vi "Navigation_Main_r1.1(new math for dist calc).vi"() -> ()   [LabVIEW 2015]
uses:
  <vilib>/myRIO/Common/Instrument Driver Framework/Utilities/typedefs/Generic FPGA Reference.ctl
  <vilib>/myRIO/Common/Instrument Driver Framework/Utilities/typedefs/myRIO v1.0 Reference.ctl
  <vilib>/myRIO/Common/Instrument Driver Framework/Utilities/typedefs/Hardware Version Enum.ctl
  <vilib>/myRIO/Common/Instrument Driver Framework/Utilities/typedefs/myRIO Generic Hardware Reference.ctl
  <vilib>/userdefined/High Color/nirio_resource_hc.ctl
  <vilib>/myRIO/Instrument Drivers/Onboard IO/PWM/typedefs/PWM Configuration.ctl
  <vilib>/myRIO/Instrument Drivers/Onboard IO/PWM/PWM.lvlib
  <vilib>/myRIO/Common/Instrument Driver Framework/myRIO v1.0/PWM/typedefs/PWM Channels Enum.ctl
  <vilib>/myRIO/Instrument Drivers/Onboard IO/PWM/typedefs/PWM Reference.ctl
  <vilib>/myRIO/Instrument Drivers/Onboard IO/PWM/vis/myRIO PWM Open.xnode
  <vilib>/myRIO/Common/Instrument Driver Framework/myRIO v1.0/PWM/vis/myRIO v1.1 Open PWM.vi
  <vilib>/rvi/interface/nirviOpenFPGA/nirviOpenFPGA.xnode
  <vilib>/myRIO/Instrument Drivers/Utilities/Utilities.lvlib
  <vilib>/rvi/interface/nirviReadWriteControl/nirviReadWriteControl.xnode
  NiFpgaLv.dll
  <vilib>/Utility/error.llb/Error Cluster From Error Code.vi
  <vilib>/rvi/interface/Simulation/niFpgaSimulationCallBeginRW.vi
  <vilib>/rvi/errors/niLvFpgaAdjustHostInterfaceError.vi
  Navi/E/FPGA Bitfiles/NavigationProjec_FPGATarget2_FPGAMainNavigati_PWPHW8gwDxI.lvbitx
  <vilib>/FPGAPlugInAG/myRIO-1900/niLvFpga_Open_myRIO-1900.vi
  <vilib>/rvi/interface/common/dynamic/niFpgaDynamicAddResources.vi
panel:
  out "x traveled":dbl
  out "x position camera":dbl
  out "x delta":dbl
  out "total":dbl
  out "step":dbl
  out "loc_flag":bool
  out "loc_x":dbl
  out "max v":dbl
  out "v left wheel":dbl
  out "v right wheel":dbl
  out "Phi desired":dbl
  out "Omega":dbl format="%.2f"
  in  "Goal Position Y":dbl=5.0
  out "x traveled":dbl
  out "y position":dbl
  out "Scale":dbl=1.0
  out "Reset X Y":dbl
  out "Desired Velocity":dbl
  out "track width(ft)":dbl=4.0
  out "phi current":dbl
  out "robot desired velocity x component\n u1 (ft/s)":dbl
  out "robot desired velocity y component\n u2 (ft/s)":dbl
  out "RM Distance (ft)":dbl
  out "RR Distance (ft)":dbl
  out "LF Distance (ft)":dbl
  out "LM Distance (ft)":dbl
  out "RF Distance (ft)":dbl
  out "LR Distance (ft)":dbl
  out "Tick Count(mSec) 2":u32 caption="Tick Count(mSec)"
  out "Right Setpoint":dbl
  out "Left Setpoint":dbl
  in  "Start Position Y":dbl=5.0
  in  "Goal Position X":dbl=5.0
  in  "Start Position X":dbl=1.0
  in  "All Stop":bool
  in  "Left Side PID Gains":T1={"proportional gain (Kc)"=0.002, "integral time (Ti, min)"=7e-07, "derivative time (Td, min)"=0.0} {"derivative time (Td, min)" format="%.8f"; "integral time (Ti, min)" format="%.8f"; "proportional gain (Kc)" format="%.8f"}
  in  "Left Side Output Range":cluster{"output high":dbl, "output low":dbl}={"output high"=0.13333, "output low"=-0.13333} {"output low" format="%.5f"; "output high" format="%.5f"}
  in  "Right Side PID Gains":T1={"proportional gain (Kc)"=0.002, "integral time (Ti, min)"=7e-07, "derivative time (Td, min)"=0.0} {"derivative time (Td, min)" format="%.8f"; "integral time (Ti, min)" format="%.8f"; "proportional gain (Kc)" format="%.8f"}
  in  "Right Side Output Range":cluster{"output high":dbl, "output low":dbl}={"output high"=0.13333, "output low"=-0.13333} {"output low" format="%.5f"; "output high" format="%.5f"}
  out "Left PWM":dbl
  out "Right PWM":dbl
  out "LF Rot Velocity (rot/s)":dbl
  out "LM Rot Velocity (rot/s)":dbl
  out "LR Rot Velocity (rot/s)":dbl
  out "RR Rot Velocity (rot/s)":dbl
  out "RM Linear Velocity (rot/s)":dbl
  out "RF Linear Velocity (rot/s)":dbl
  in  "Encoder Reset":bool
  out "SYS.SELECTA":u8 format="%08b"
  out "ENC.B_c.CNTR":i32
  out "ENC.B_b.CNTR":i32
  out "ENC.B_a.CNTR":i32
  out "ENC.A_c.CNTR":i32
  out "ENC.A_b.CNTR":i32
  out "ENC.A_a.CNTR":i32
  out "Current Rot Velocity (rot/s)":T2(graph)
  # "Motor Control Parameters"
  # "Press Go when Start and Goal Are Set"
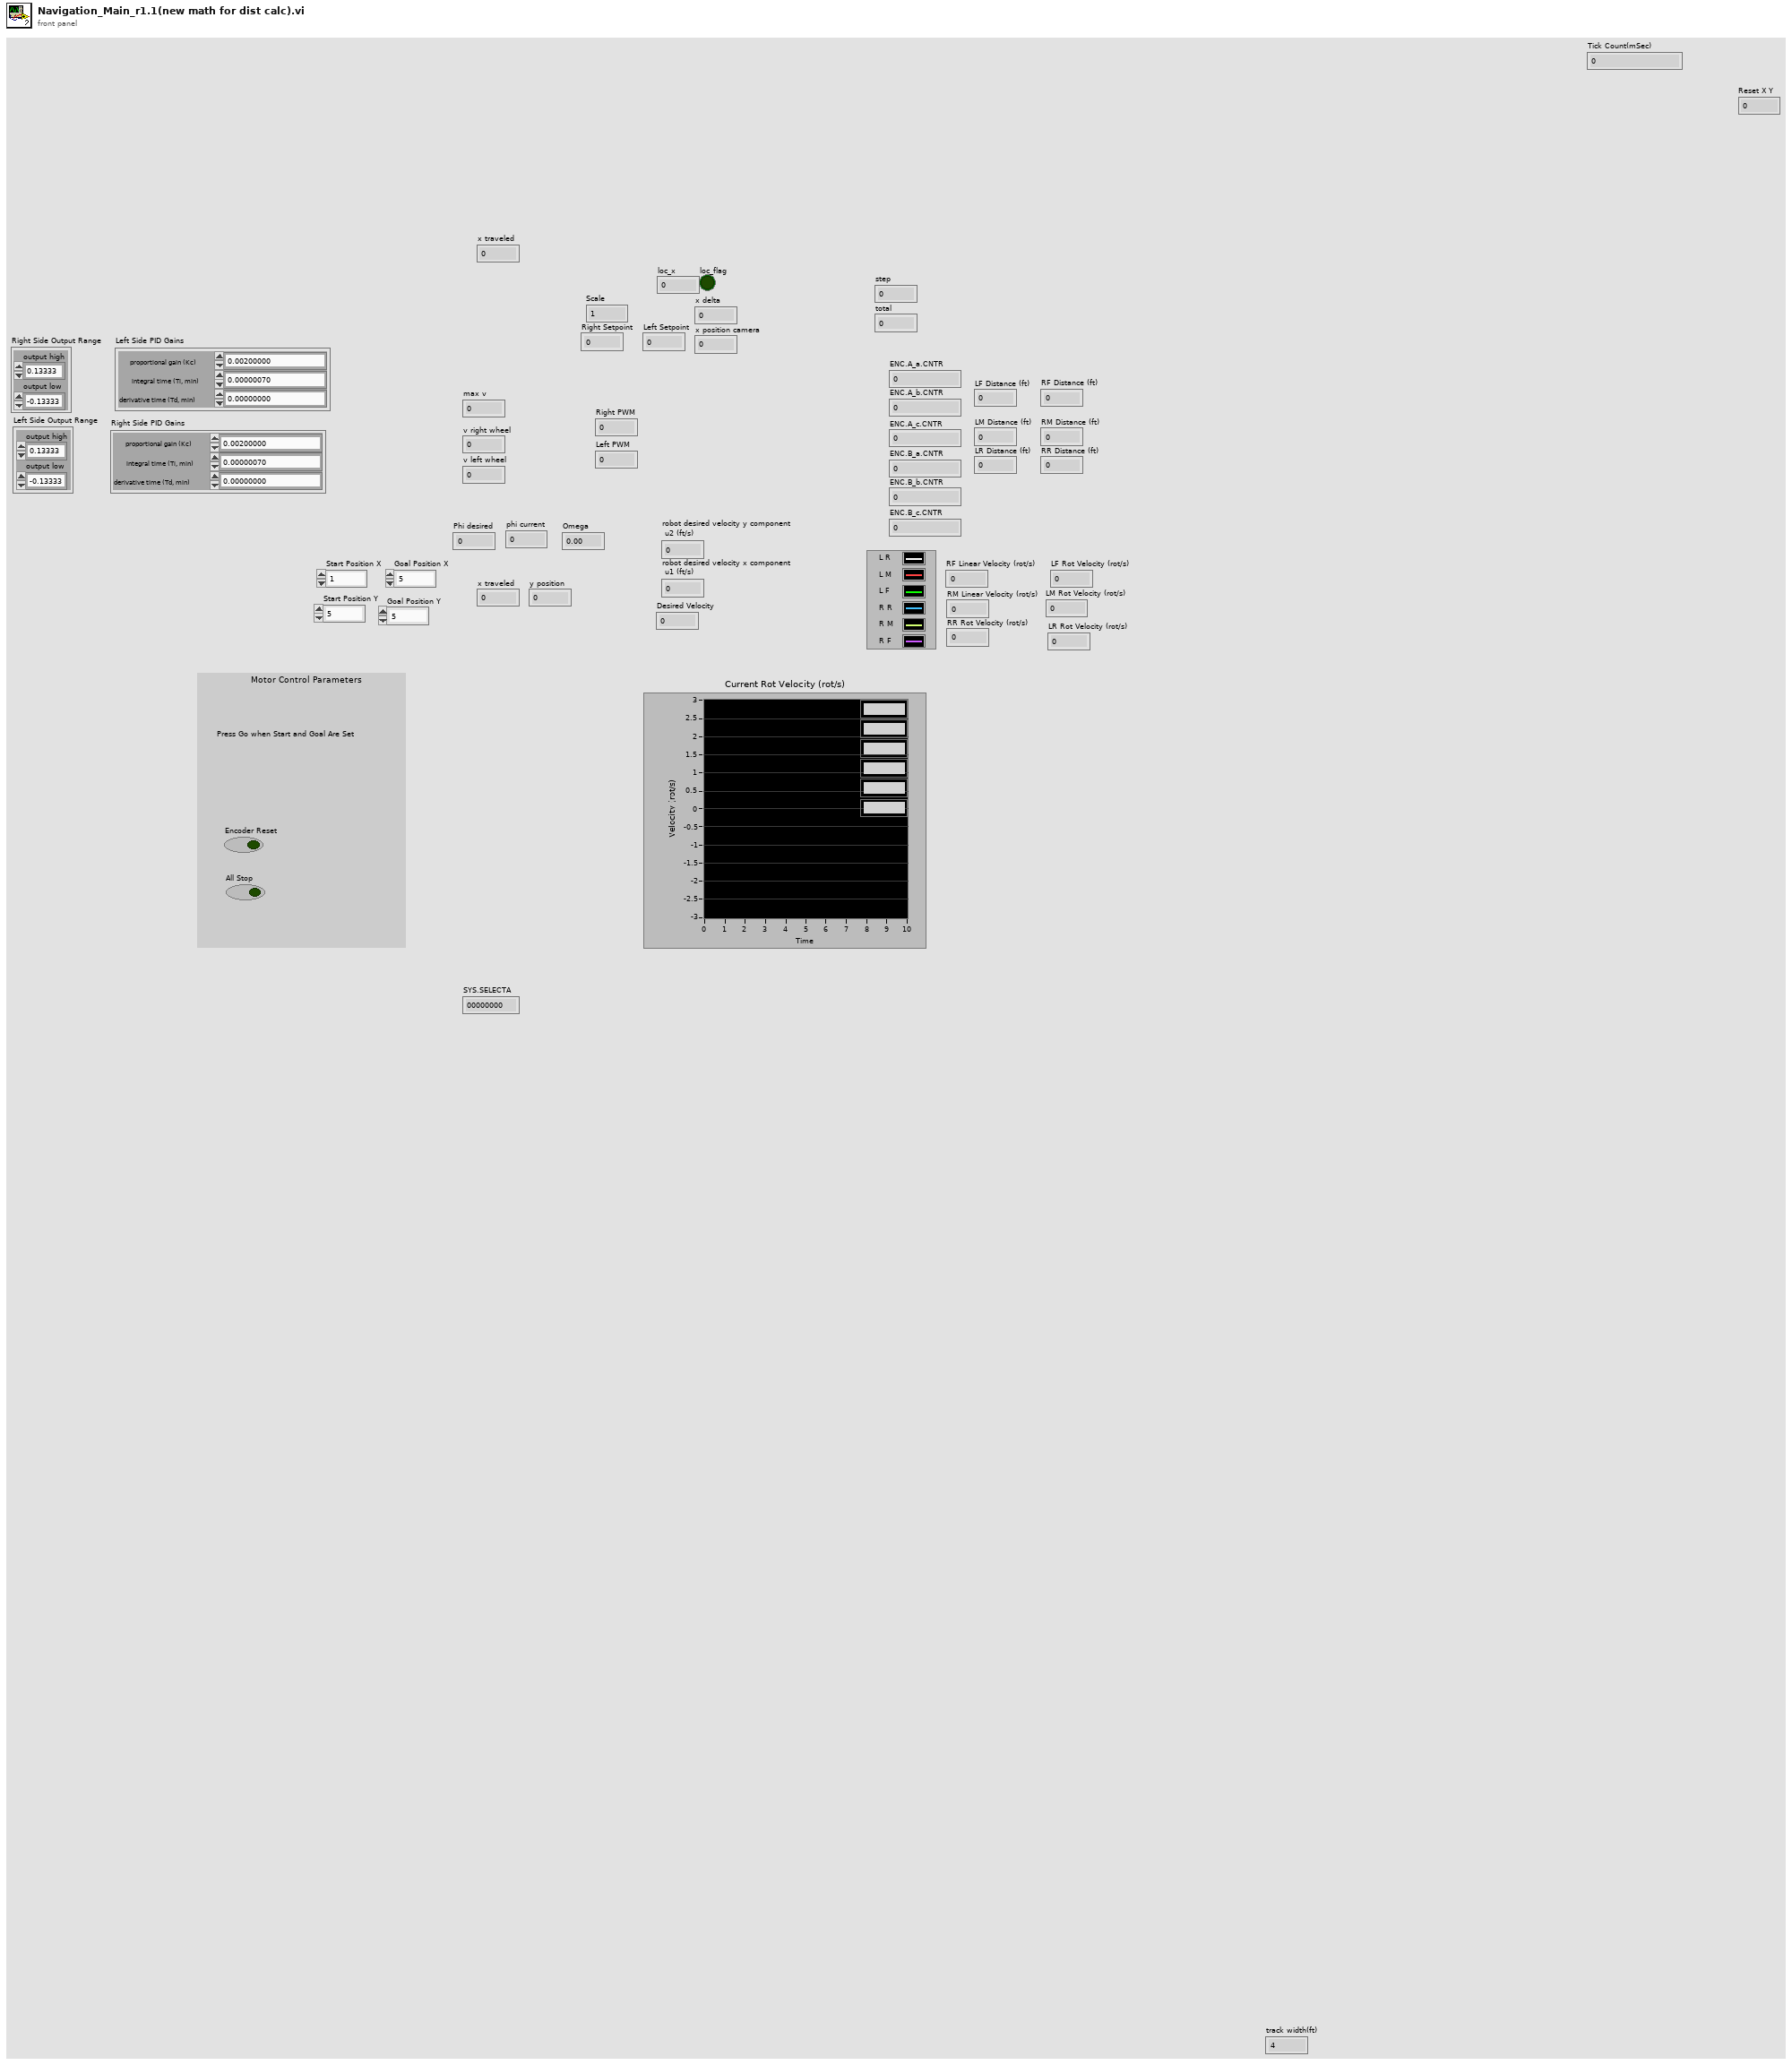
[diagram p1: front panel]
types:
  T1 = cluster{"proportional gain (Kc)":dbl, "integral time (Ti, min)":dbl, "derivative time (Td, min)":dbl}
  T2 = cluster{"Rotational Velocity (RPS)":dbl, "Rotational Velocity (RPS)":dbl, "Rotational Velocity (RPS)":dbl, "Rotational Velocity (RPS)":dbl, "Rotational Velocity (RPS)":dbl, "Rotational Velocity (RPS)":dbl}
  T3 = typedef "nirio_resource_hc.ctl" = tag
  T4 = typedef "Hardware Version Enum.ctl" = enum16{"Unknown", "myRIO-1900", "myRIO-1950", "roboRIO"}
  T5 = typedef "PWM.lvlib/PWM Reference.ctl" = cluster{"myRIO Reference":T6, "PWM Channels Enum":T9, "PWM Configuration":T10}
  T6 = typedef "myRIO Generic Hardware Reference.ctl" = cluster{"myRIO Model":T4, "myRIO Hardware Reference":T7}
  T7 = typedef "myRIO v1.0 Reference.ctl" = cluster{"Generic FPGA Reference":T8, "Allow multiple opens":bool}
  T8 = typedef "Generic FPGA Reference.ctl" = refnum<k20>
  T9 = typedef "PWM Channels Enum.ctl" = enum16{"Not Connected", "C/PWM0", "C/PWM1", "A/PWM0", "A/PWM1", "A/PWM2", "B/PWM0", "B/PWM1", "B/PWM2", "PWM/PWM0", "PWM/PWM1", "PWM/PWM2", "PWM/PWM3", "PWM/PWM4", "PWM/PWM5", "PWM/PWM6", "PWM/PWM7", "PWM/PWM8", "PWM/PWM9"}
  T10 = typedef "PWM.lvlib/PWM Configuration.ctl" = cluster{"Frequency":dbl, "Duty Cycle":dbl}
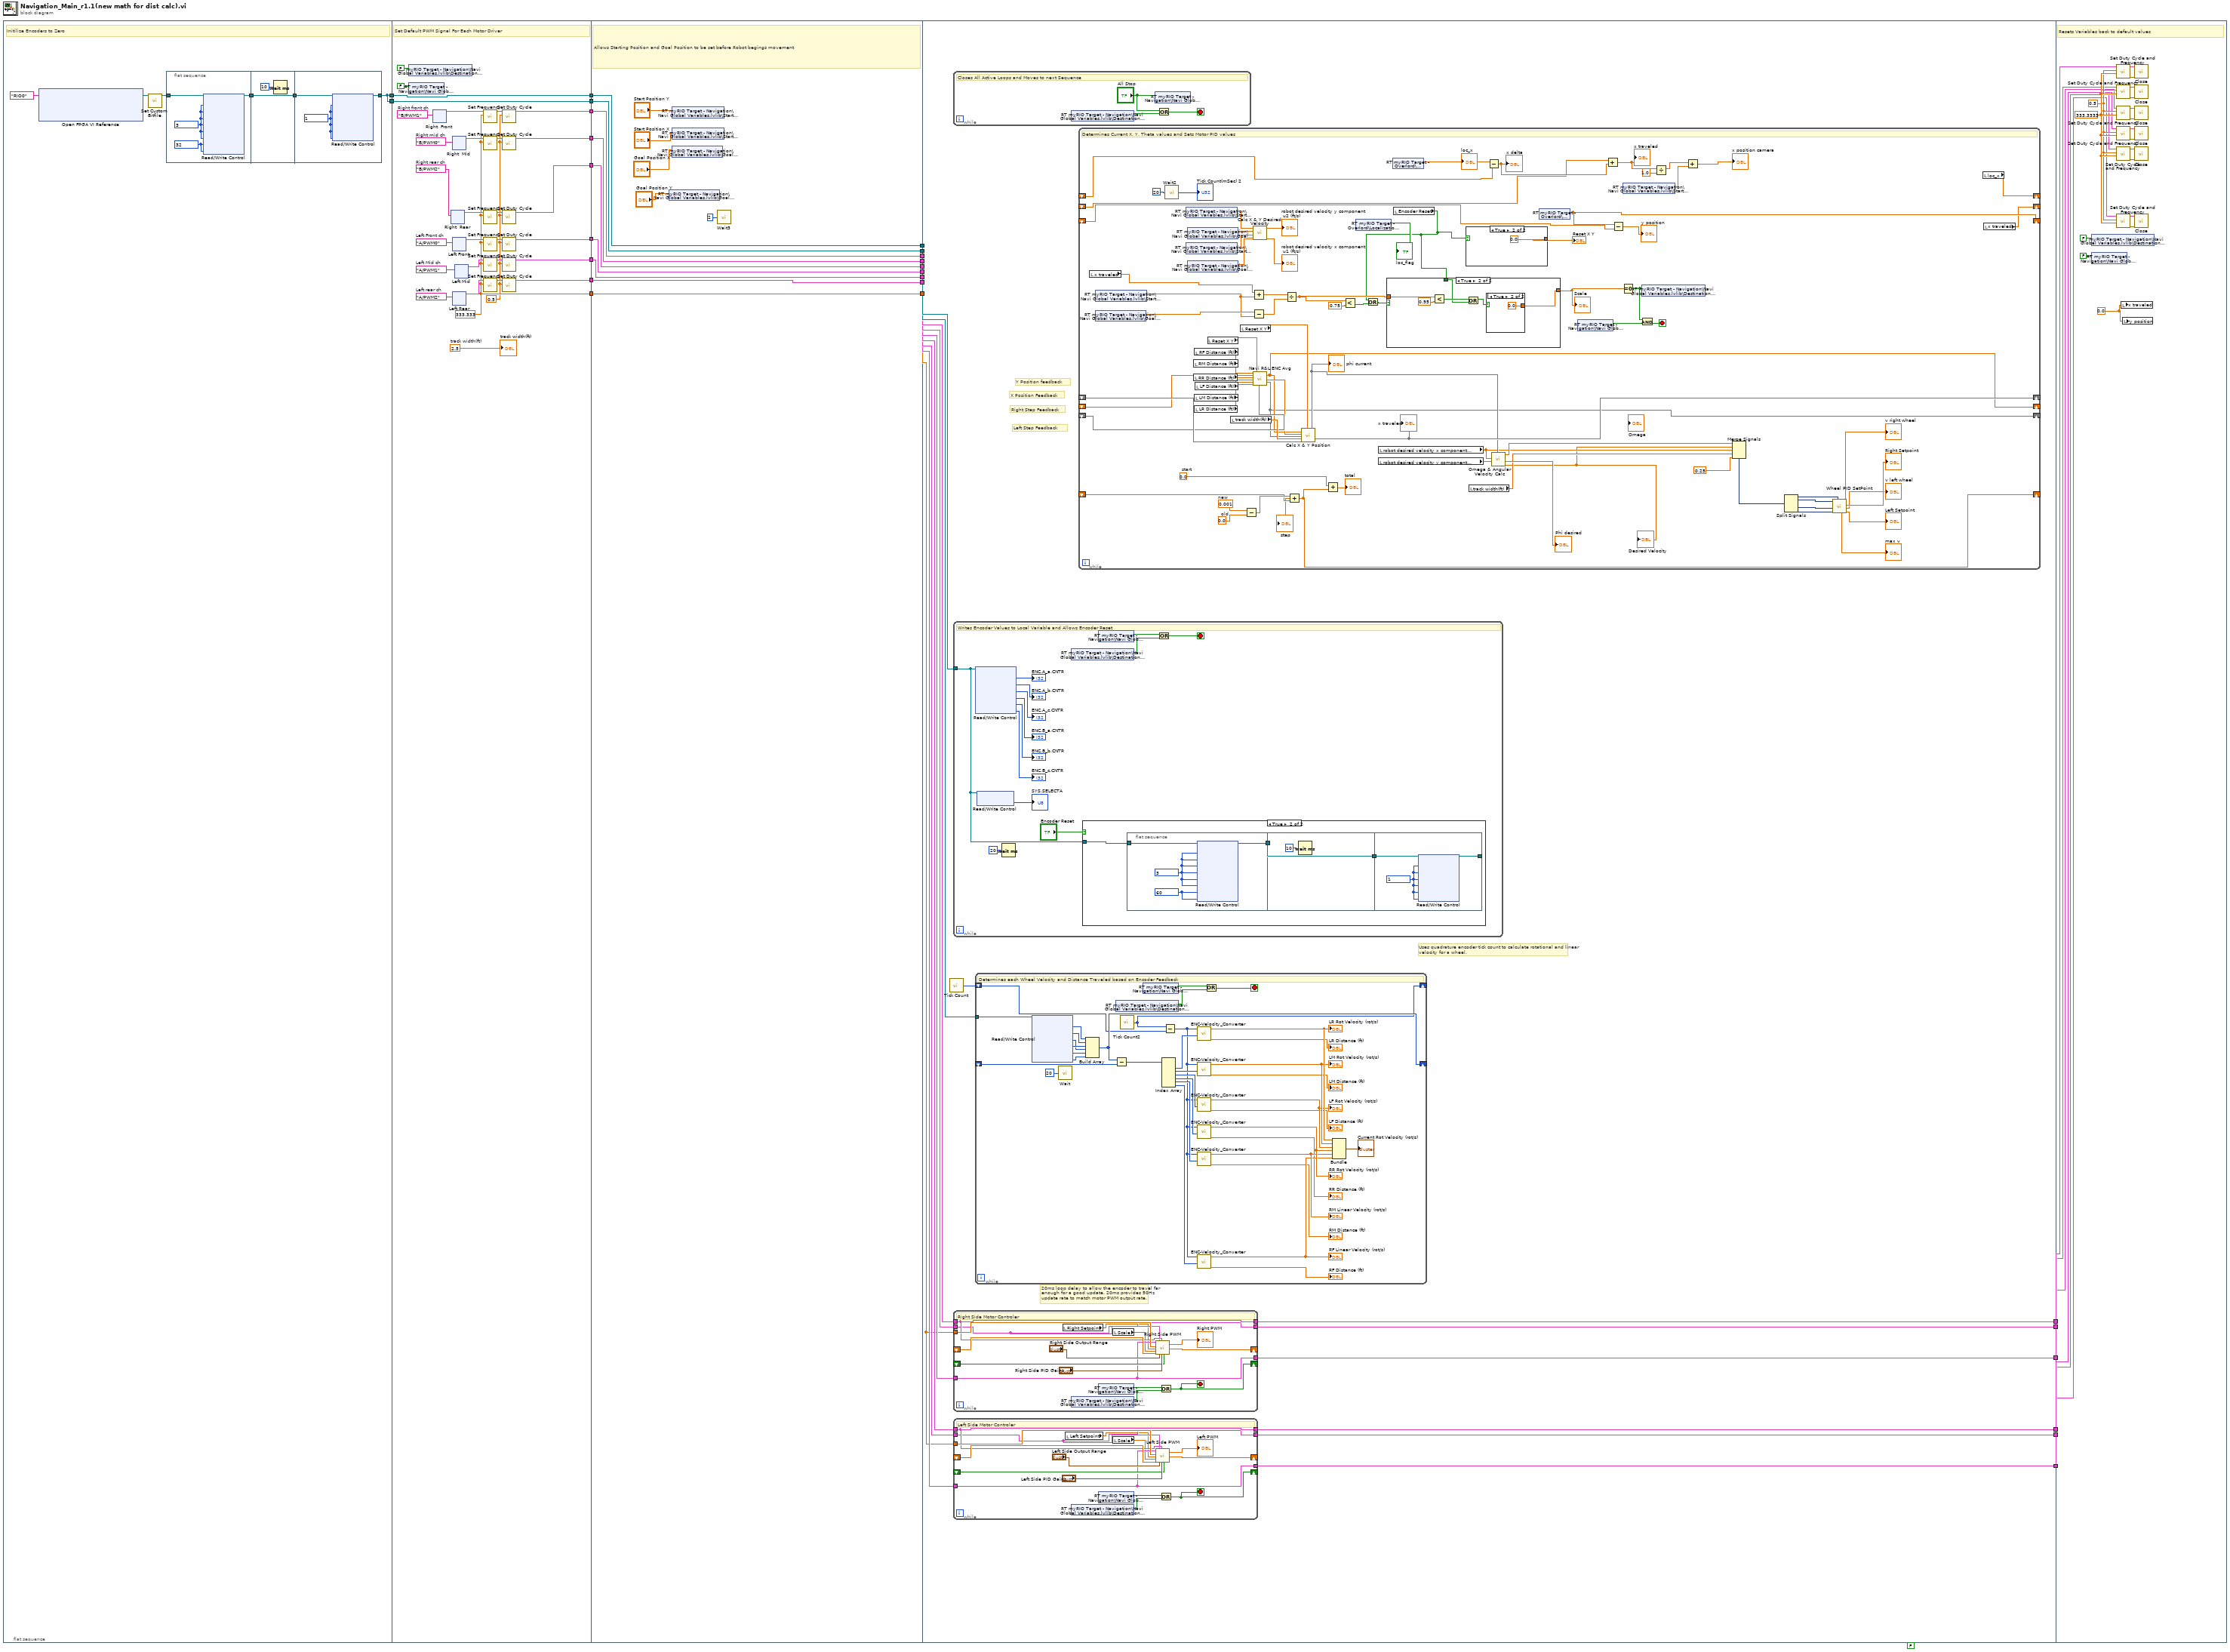
[diagram p0: block diagram]
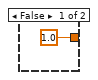
[diagram p2: hidden frame]
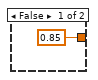
[diagram p3: hidden frame]
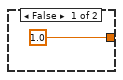
[diagram p4: hidden frame]
diagram:
  (unwired) FALSE ("stop")
  n1 = flat-sequence {
    tunnel: [w29] -> w26
    tunnel: [w29] -> w25
    tunnel: [w60] -> w24
    tunnel: [w55] -> w23
    tunnel: [w51] -> w22
    tunnel: [w50] -> w21
    tunnel: [w49] -> w20
    tunnel: [w48] -> w19
    tunnel: [w47] -> w18
    tunnel: [w46] -> w17
    tunnel: w26 -> [w45]
    tunnel: [w45] -> w16
    tunnel: w25 -> [w46]
    tunnel: w24 -> [w182]
    tunnel: [w182] -> w15
    tunnel: w23 -> [w181]
    tunnel: [w181] -> w14
    tunnel: w22 -> [w180]
    tunnel: [w180] -> w13
    tunnel: w21 -> [w179]
    tunnel: [w179] -> w12
    tunnel: w20 -> [w178]
    tunnel: [w178] -> w11
    tunnel: w19 -> [w177]
    tunnel: [w177] -> w10
    tunnel: w18 -> [w176]
    tunnel: [w176] -> w9
    tunnel: w17 -> [w175]
    tunnel: [w175] -> w8
    tunnel: w16 -> [w174]
    tunnel: [w174] -> w7
    tunnel: w15 -> [w189]
    tunnel: w14 -> [w190]
    tunnel: w13 -> [w195]
    tunnel: w12 -> [w194]
    tunnel: w11 -> [w193]
    tunnel: w10 -> [w192]
    tunnel: w9 -> [w191]
    tunnel: w8 -> [w197]
    tunnel: w7 -> [w196]
    tunnel: [w188] -> w6
    tunnel: [w187] -> w5
    tunnel: [w186] -> w4
    tunnel: [w185] -> w3
    tunnel: [w184] -> w2
    tunnel: [w183] -> w1
    tunnel: w6 -> [w391]
    tunnel: w5 -> [w390]
    tunnel: w4 -> [w389]
    tunnel: w3 -> [w388]
    tunnel: w2 -> [w387]
    tunnel: w1 -> [w386]
    frame #0 {
      # "Initilize Encoders to Zero"
      n2 = xnode "Open FPGA VI Reference"("resource name"=tag "RIO0") -> ("FPGA VI Reference Out"=w28:refnum<k20>)  [unwired: 1 in, 1 out]
      n3 = call <vilib>:"Set Custom Bitfile.vi"("Custom FPGA Reference In"=w28) -> ("Custom FPGA Reference Out"=w30:refnum<k20>)  [unwired: 9 in, 1 out]
      n4 = flat-sequence {
        tunnel: w30 -> [w35]
        tunnel: [w33] -> w32
        tunnel: w32 -> [w37]
        tunnel: [w37] -> w31
        tunnel: w31 -> [w40]
        tunnel: [w39] -> w29
        frame #0 {
          w34 = u8 32 ("SYS.SELECTA")
          w36 = u8 3 ("ENC.B_c.CNFG")
          n5 = xnode "Read/Write Control"("FPGA VI Reference In"=w35, "ENC.A_a.CNFG"=w36, "ENC.A_b.CNFG"=w36, "ENC.A_c.CNFG"=w36, "ENC.B_a.CNFG"=w36, "ENC.B_b.CNFG"=w36, "ENC.B_c.CNFG"=w36, "SYS.SELECTA"=w34, "SYS.SELECTB"=w34) -> ("FPGA VI Reference Out"=w33:refnum<k20>)  [unwired: 1 in, 1 out]
        }
        frame #1 {
          n6 = Wait (ms)(milliseconds to wait=u32 10) -> ()  [unwired: 1 out]
        }
        frame #2 {
          w41 = u8 1 ("ENC.B_c.CNFG")
          n7 = xnode "Read/Write Control"("FPGA VI Reference In"=w40, "ENC.A_a.CNFG"=w41, "ENC.A_b.CNFG"=w41, "ENC.A_c.CNFG"=w41, "ENC.B_a.CNFG"=w41, "ENC.B_b.CNFG"=w41, "ENC.B_c.CNFG"=w41) -> ("FPGA VI Reference Out"=w39:refnum<k20>)  [unwired: 1 in, 1 out]
        }
      }
    }
    frame #1 {
      w42 = 2.5  # track width(ft)
      w52 = 0.5 ("Duty Cycle")
      w60 = 333.333 ("Frequency [Hz]")
      w67 = tag "B/PWM2"  # Right rear ch
      w68 = tag "B/PWM0"  # Right mid ch
      w69 = tag "B/PWM1"  # Right front ch
      w70 = tag "A/PWM2"  # Left rear ch
      w71 = tag "A/PWM0"  # Left Front ch
      w72 = tag "A/PWM1"  # Left Mid ch
      # "Set Default PWM Signal For Each Motor Driver"
      n8 = shared-variable "RT myRIO Target - Navigation\\Navi Global Variables.lvlib\\Destination Reached"(FALSE) -> ()  [unwired: 1 in, 1 out]
      n9 = shared-variable "RT myRIO Target - Navigation\\Navi Global Variables.lvlib\\All Stop"(FALSE) -> ()  [unwired: 1 in, 1 out]
      n10 = xnode "Right  Front"("Channel Name"=w69) -> ("PWM Ref Out"=w63:T5)  [unwired: 2 in, 1 out]
      n11 = xnode "Right  Rear"("Channel Name"=w67) -> ("PWM Ref Out"=w61:T5)  [unwired: 2 in, 1 out]
      n12 = xnode "Right  Mid"("Channel Name"=w68) -> ("PWM Ref Out"=w62:T5)  [unwired: 2 in, 1 out]
      n13 = xnode "Left Front"("Channel Name"=w71) -> ("PWM Ref Out"=w65:T5)  [unwired: 2 in, 1 out]
      n14 = xnode "Left Rear"("Channel Name"=w70) -> ("PWM Ref Out"=w64:T5)  [unwired: 2 in, 1 out]
      n15 = xnode "Left Mid"("Channel Name"=w72) -> ("PWM Ref Out"=w66:T5)  [unwired: 2 in, 1 out]
      n16 = call <vilib>:"Set Frequency.vi"("Frequency [Hz]"=w60, "PWM Ref In"=w63) -> ("PWM Ref Out"=w56:T5)  [unwired: 7 in, 1 out]
      n17 = call <vilib>:"Set Frequency.vi"("Frequency [Hz]"=w60, "PWM Ref In"=w62) -> ("PWM Ref Out"=w57:T5)  [unwired: 7 in, 1 out]
      n18 = call <vilib>:"Set Frequency.vi"("Frequency [Hz]"=w60, "PWM Ref In"=w61) -> ("PWM Ref Out"=w58:T5)  [unwired: 7 in, 1 out]
      n19 = call <vilib>:"Set Frequency.vi"("Frequency [Hz]"=w60, "PWM Ref In"=w65) -> ("PWM Ref Out"=w53:T5)  [unwired: 7 in, 1 out]
      n20 = call <vilib>:"Set Frequency.vi"("Frequency [Hz]"=w60, "PWM Ref In"=w66) -> ("PWM Ref Out"=w59:T5)  [unwired: 7 in, 1 out]
      n21 = call <vilib>:"Set Frequency.vi"("Frequency [Hz]"=w60, "PWM Ref In"=w64) -> ("PWM Ref Out"=w54:T5)  [unwired: 7 in, 1 out]
      n22 = call <vilib>:"Set Duty Cycle.vi"("Duty Cycle"=w52, "PWM Ref In"=w56) -> ("PWM Ref Out"=w51:T5)  [unwired: 7 in, 1 out]
      n23 = call <vilib>:"Set Duty Cycle.vi"("Duty Cycle"=w52, "PWM Ref In"=w57) -> ("PWM Ref Out"=w50:T5)  [unwired: 7 in, 1 out]
      n24 = call <vilib>:"Set Duty Cycle.vi"("Duty Cycle"=w52, "PWM Ref In"=w58) -> ("PWM Ref Out"=w49:T5)  [unwired: 7 in, 1 out]
      n25 = call <vilib>:"Set Duty Cycle.vi"("Duty Cycle"=w52, "PWM Ref In"=w53) -> ("PWM Ref Out"=w48:T5)  [unwired: 7 in, 1 out]
      n26 = call <vilib>:"Set Duty Cycle.vi"("Duty Cycle"=w52, "PWM Ref In"=w59) -> ("PWM Ref Out"=w47:T5)  [unwired: 7 in, 1 out]
      n27 = call <vilib>:"Set Duty Cycle.vi"("Duty Cycle"=w52, "PWM Ref In"=w54) -> ("PWM Ref Out"=w55:T5)  [unwired: 7 in, 1 out]
      "track width(ft)" <- w42
    }
    frame #2 {
      # "Allows Starting Position and Goal Position to be set before Robot begings movement"
      n28 = shared-variable "RT myRIO Target - Navigation\\Navi Global Variables.lvlib\\Goal Position Y"("Goal Position Y") -> ()  [unwired: 1 in, 1 out]
      n29 = shared-variable "RT myRIO Target - Navigation\\Navi Global Variables.lvlib\\Start Position Y"("Start Position Y") -> ()  [unwired: 1 in, 1 out]
      n30 = shared-variable "RT myRIO Target - Navigation\\Navi Global Variables.lvlib\\Start Position X"("Start Position X") -> ()  [unwired: 1 in, 1 out]
      n31 = shared-variable "RT myRIO Target - Navigation\\Navi Global Variables.lvlib\\Goal Position X"("Goal Position X") -> ()  [unwired: 1 in, 1 out]
      n32 = call "Wait3"("Count(mSec)"=u32 2) -> ()  [unwired: 1 out]
    }
    frame #3 {
      # "Left Step Feedback"
      # "Y Position feedback"
      # "Right Step Feedback"
      # "X Position Feedback"
      # "Uses quadrature encoder tick count to calculate rotational and linear velocity for a wheel."
      # "20ms loop delay to allow the encoder to travel far enough for a good update. 20ms provides 50Hz update rate to match motor PWM output rate."
      n33 = call "Tick Count"() -> ("Tick Count(uSec)"=w198:u32)
      n34 = while {
        stop <- w291 stop-if-true
        # "Closes All Active Loops and Moves to next Sequence"
        n35 = shared-variable "RT myRIO Target - Navigation\\Navi Global Variables.lvlib\\Destination Reached"() -> (w289:bool)  [unwired: 1 in, 1 out]
        n36 = shared-variable "RT myRIO Target - Navigation\\Navi Global Variables.lvlib\\All Stop"("All Stop") -> ()  [unwired: 1 in, 1 out]
        n37 = Or(x="All Stop", y=w289) -> (x .or. y?=w291:bool)
      }
      n38 = while {
        tunnel: w197 -> [w325]
        stop <- w322 stop-if-true
        # "Writes Encoder Values to Local Variable and Allows Encoder Reset"
        n39 = xnode "Read/Write Control"("FPGA VI Reference In"=w325) -> ("ENC.A_a.CNTR"=→"ENC.A_a.CNTR":u32, "ENC.A_b.CNTR"=→"ENC.A_b.CNTR":u32, "ENC.A_c.CNTR"=→"ENC.A_c.CNTR":u32, "ENC.B_a.CNTR"=→"ENC.B_a.CNTR":u32, "ENC.B_b.CNTR"=→"ENC.B_b.CNTR":u32, "ENC.B_c.CNTR"=→"ENC.B_c.CNTR":u32)  [unwired: 1 in, 2 out]
        n40 = xnode "Read/Write Control"("FPGA VI Reference In"=w325) -> ("SYS.SELECTA"=→"SYS.SELECTA":u8)  [unwired: 1 in, 2 out]
        n41 = Wait (ms)(milliseconds to wait=u32 20) -> ()  [unwired: 1 out]
        n42 = shared-variable "RT myRIO Target - Navigation\\Navi Global Variables.lvlib\\Destination Reached"() -> (w324:bool)  [unwired: 1 in, 1 out]
        n43 = case shown="True" "Encoder Reset" {
          tunnel: w325 -> [_ w335]
          frame False {
          }
          frame True {
            n44 = flat-sequence {
              tunnel: w335 -> [w340]
              tunnel: [w338] -> w337
              tunnel: w337 -> [w342]
              tunnel: [w342] -> w336
              tunnel: w336 -> [w345]
              tunnel: [w344] -> _
              frame #0 {
                w339 = u8 60 ("SYS.SELECTA")
                w341 = u8 3 ("ENC.B_c.CNFG")
                n45 = xnode "Read/Write Control"("FPGA VI Reference In"=w340, "ENC.A_a.CNFG"=w341, "ENC.A_b.CNFG"=w341, "ENC.A_c.CNFG"=w341, "ENC.B_a.CNFG"=w341, "ENC.B_b.CNFG"=w341, "ENC.B_c.CNFG"=w341, "SYS.SELECTA"=w339, "SYS.SELECTB"=w339) -> ("FPGA VI Reference Out"=w338:refnum<k20>)  [unwired: 1 in, 1 out]
              }
              frame #1 {
                n46 = Wait (ms)(milliseconds to wait=u32 10) -> ()  [unwired: 1 out]
              }
              frame #2 {
                w346 = u8 1 ("ENC.B_c.CNFG")
                n47 = xnode "Read/Write Control"("FPGA VI Reference In"=w345, "ENC.A_a.CNFG"=w346, "ENC.A_b.CNFG"=w346, "ENC.A_c.CNFG"=w346, "ENC.B_a.CNFG"=w346, "ENC.B_b.CNFG"=w346, "ENC.B_c.CNFG"=w346) -> ("FPGA VI Reference Out"=w344:refnum<k20>)  [unwired: 1 in, 1 out]
              }
            }
          }
        }
        n48 = shared-variable "RT myRIO Target - Navigation\\Navi Global Variables.lvlib\\All Stop"() -> (w323:bool)  [unwired: 1 in, 1 out]
        n49 = Or(x=w323, y=w324) -> (x .or. y?=w322:bool)
      }
      n50 = while {
        tunnel: w195 -> [w314]
        tunnel: w194 -> [w313]
        tunnel: w193 -> [w312]
        tunnel: w189 -> [w321]
        shift-right: [w317] -> _
        shift-left: _ -> [w316]
        shift-right: [w309] -> _
        shift-left: _ -> [w315]
        tunnel: [w314] -> w188
        tunnel: [w313] -> w187
        tunnel: [w312] -> w186
        stop <- w309 stop-if-true
        # "Right Side Motor Controler"
        n51 = local read "Right Setpoint"() -> (w308:dbl)
        n52 = shared-variable "RT myRIO Target - Navigation\\Navi Global Variables.lvlib\\Destination Reached"() -> (w311:bool)  [unwired: 1 in, 1 out]
        n53 = shared-variable "RT myRIO Target - Navigation\\Navi Global Variables.lvlib\\All Stop"() -> (w310:bool)  [unwired: 1 in, 1 out]
        n54 = local read "Scale"() -> (w307:dbl)
        n55 = call "Right Side PWM.vi"("Right rear"=w312, "Frequency"=w321, "Right Side Setpoint"=w308, "Right Side Scale"=w307, "Right PID Feedback"=w316, "Right Mid"=w313, "Right Side Output Range"="Right Side Output Range", "Right Front"=w314, "Right Side PID Gains"="Right Side PID Gains", "Reset Right E.T."=w315) -> ("Right PWM"=→"Right PWM":dbl, "Right PID Output"=w317:dbl)  [unwired: 8 in]
        n56 = Or(x=w310, y=w311) -> (x .or. y?=w309:bool)
      }
      n57 = while {
        tunnel: w192 -> [w299]
        tunnel: w191 -> [w298]
        tunnel: w190 -> [w297]
        tunnel: w189 -> [w306]
        shift-right: [w302] -> _
        shift-left: _ -> [w301]
        shift-right: [w294] -> _
        shift-left: _ -> [w300]
        tunnel: [w299] -> w185
        tunnel: [w298] -> w184
        tunnel: [w297] -> w183
        stop <- w294 stop-if-true
        # "Left Side Motor Controler"
        n58 = local read "Left Setpoint"() -> (w293:dbl)
        n59 = shared-variable "RT myRIO Target - Navigation\\Navi Global Variables.lvlib\\Destination Reached"() -> (w296:bool)  [unwired: 1 in, 1 out]
        n60 = shared-variable "RT myRIO Target - Navigation\\Navi Global Variables.lvlib\\All Stop"() -> (w295:bool)  [unwired: 1 in, 1 out]
        n61 = local read "Scale"() -> (w292:dbl)
        n62 = call "Left Side PWM.vi"("Left rear"=w297, "Frequency"=w306, "Left Side Setpoint"=w293, "Left Side Scale"=w292, "Left PID Feedback"=w301, "Left Mid"=w298, "Left Side Output Range"="Left Side Output Range", "Left Front"=w299, "Left Side PID Gains"="Left Side PID Gains", "Reset Left E.T."=w300) -> ("Left PWM"=→"Left PWM":dbl, "Left PID Output"=w302:dbl)  [unwired: 8 in]
        n63 = Or(x=w295, y=w296) -> (x .or. y?=w294:bool)
      }
      n64 = while {
        shift-right: [w374] -> _
        shift-left: _ -> [w373]
        shift-right: [w371] -> _
        shift-left: w198 -> [w370]
        tunnel: w196 -> [w381]
        stop <- w366 stop-if-true
        # "Determines each Wheel Velocity and Distance Traveled based on Encoder Feedback"
        n65 = xnode "Read/Write Control"("FPGA VI Reference In"=w381) -> ("ENC.A_a.CNTR"=w380:u32, "ENC.A_b.CNTR"=w379:u32, "ENC.A_c.CNTR"=w378:u32, "ENC.B_a.CNTR"=w377:u32, "ENC.B_b.CNTR"=w376:u32, "ENC.B_c.CNTR"=w375:u32)  [unwired: 1 in, 2 out]
        n66 = call "Wait"("Count(mSec)"=u32 20) -> ()  [unwired: 1 out]
        n67 = Build Array(w380, w379, w378, w377, w376, w375) -> (w374:u32[])
        n68 = Subtract(x=w374, y=w373) -> (x-y=w372:u32[])
        n69 = shared-variable "RT myRIO Target - Navigation\\Navi Global Variables.lvlib\\Destination Reached"() -> (w368:bool)  [unwired: 1 in, 1 out]
        n70 = call "Tick Count2"() -> ("Tick Count(uSec)"=w371:u32)
        n71 = shared-variable "RT myRIO Target - Navigation\\Navi Global Variables.lvlib\\All Stop"() -> (w367:bool)  [unwired: 1 in, 1 out]
        n72 = Index Array(array=w372) -> (element #1=w365:u32, element #2=w362:u32, element #3=w360:u32, element #4=w358:u32, element #5=w356:u32, element #6=w353:u32)  [unwired: 6 in]
        n73 = Subtract(x=w371, y=w370) -> (x-y=w354:u32)
        n74 = call "ENC-Velocity_Converter.vi"("delta  Encoder Count"=w365, "dt (uSec)"=w354) -> ("Distance (ft)"=→"LR Distance (ft)":dbl, "Rotational Velocity (RPS)"=w364:dbl)  [unwired: 7 in, 1 out]
        "LR Rot Velocity (rot/s)" <- w364
        n75 = call "ENC-Velocity_Converter.vi"("delta  Encoder Count"=w362, "dt (uSec)"=w354) -> ("Distance (ft)"=→"LM Distance (ft)":dbl, "Rotational Velocity (RPS)"=w363:dbl)  [unwired: 7 in, 1 out]
        "LM Rot Velocity (rot/s)" <- w363
        n76 = call "ENC-Velocity_Converter.vi"("delta  Encoder Count"=w360, "dt (uSec)"=w354) -> ("Distance (ft)"=→"LF Distance (ft)":dbl, "Rotational Velocity (RPS)"=w361:dbl)  [unwired: 7 in, 1 out]
        "LF Rot Velocity (rot/s)" <- w361
        n77 = call "ENC-Velocity_Converter.vi"("delta  Encoder Count"=w358, "dt (uSec)"=w354) -> ("Distance (ft)"=→"RR Distance (ft)":dbl, "Rotational Velocity (RPS)"=w359:dbl)  [unwired: 7 in, 1 out]
        "RR Rot Velocity (rot/s)" <- w359
        n78 = call "ENC-Velocity_Converter.vi"("delta  Encoder Count"=w356, "dt (uSec)"=w354) -> ("Distance (ft)"=→"RM Distance (ft)":dbl, "Rotational Velocity (RPS)"=w357:dbl)  [unwired: 7 in, 1 out]
        "RM Linear Velocity (rot/s)" <- w357
        n79 = call "ENC-Velocity_Converter.vi"("delta  Encoder Count"=w353, "dt (uSec)"=w354) -> ("Distance (ft)"=→"RF Distance (ft)":dbl, "Rotational Velocity (RPS)"=w355:dbl)  [unwired: 7 in, 1 out]
        "RF Linear Velocity (rot/s)" <- w355
        n80 = Or(x=w367, y=w368) -> (x .or. y?=w366:bool)
        n81 = Bundle("Rotational Velocity (RPS)"=w364, "Rotational Velocity (RPS)"=w363, "Rotational Velocity (RPS)"=w361, "Rotational Velocity (RPS)"=w359, "Rotational Velocity (RPS)"=w357, "Rotational Velocity (RPS)"=w355) -> (→"Current Rot Velocity (rot/s)":T2)  [unwired: 1 in]
      }
      n82 = while {
        shift-right: [w265] -> _
        shift-left: _ -> [w266]
        shift-right: [w243] -> _
        shift-left: _ -> [w263]
        shift-right: [w218] -> _
        shift-left: _ -> [w262]
        shift-right: [w207] -> _
        shift-left: _ -> [w209]
        shift-right: [w223] -> _
        shift-left: _ -> [w224]
        shift-right: [w204] -> _
        shift-left: _ -> [w205]
        shift-right: [w214] -> _
        shift-left: _ -> [w216]
        stop <- w273 stop-if-true
        w219 = 0.0  # old
        w220 = 0.001  # new
        w215 = 0.0  # start
        # "Determines Current X, Y, Theta values and Sets Motor PID values"
        n83 = local read "x traveled"() -> (w221:dbl)
        n84 = shared-variable "RT myRIO Target - Navigation\\Navi Global Variables.lvlib\\Start Position X"() -> (w208:dbl)  [unwired: 1 in, 1 out]
        n85 = shared-variable "RT myRIO Target - Navigation\\Navi Global Variables.lvlib\\Goal Position X"() -> (w244:dbl)  [unwired: 1 in, 1 out]
        n86 = call "Wait2"("Count(mSec)"=u32 20) -> ("Tick Count(mSec)"=→"Tick Count(mSec) 2":u32)
        n87 = shared-variable "RT myRIO Target - Navigation\\Navi Global Variables.lvlib\\Start Position Y"() -> (w272:dbl)  [unwired: 1 in, 1 out]
        n88 = shared-variable "RT myRIO Target - Navigation\\Navi Global Variables.lvlib\\Start Position X"() -> (w270:dbl)  [unwired: 1 in, 1 out]
        n89 = shared-variable "RT myRIO Target - Navigation\\Navi Global Variables.lvlib\\Goal Position Y"() -> (w271:dbl)  [unwired: 1 in, 1 out]
        n90 = shared-variable "RT myRIO Target - Navigation\\Navi Global Variables.lvlib\\Goal Position X"() -> (w269:dbl)  [unwired: 1 in, 1 out]
        n91 = local read "RM Distance (ft)"() -> (w260:dbl)
        n92 = local read "RR Distance (ft)"() -> (w259:dbl)
        n93 = local read "RF Distance (ft)"() -> (w261:dbl)
        n94 = local read "LM Distance (ft)"() -> (w257:dbl)
        n95 = local read "LR Distance (ft)"() -> (w256:dbl)
        n96 = local read "LF Distance (ft)"() -> (w258:dbl)
        n97 = local read "Reset X Y"() -> (w246:dbl)
        n98 = local read "track width(ft)"() -> (w264:dbl)
        n99 = local read "Reset X Y"() -> (w245:dbl)
        n100 = Subtract(x=w220, y=w219) -> (x-y=w217:dbl)
        n101 = Add(x=w221, y=w208) -> (x+y=w249:dbl)
        n102 = Subtract(x=w244, y=w208) -> (x-y=w247:dbl)
        n103 = call "Calc X & Y Desired Velocity.vi"("x goal"=w269, "x start"=w270, "Y Goal"=w271, "Y Position"=w272) -> ("robot desired velocity x component\n u1 (ft/s)"=→"robot desired velocity x component\n u1 (ft/s)":dbl, "robot desired velocity y component\n u2 (ft/s)"=→"robot desired velocity y component\n u2 (ft/s)":dbl)  [unwired: 6 in]
        n104 = Divide(x=w249, y=w247) -> (x/y=w248:dbl)
        n105 = Add(x=w217, y=w216) -> (x+y=w214:dbl)
        "step" <- w214
        n106 = Add(x=w215, y=w214) -> (x+y=→"total":dbl)
        n107 = Less?(x=w248, y=0.75) -> (x < y?=w212:bool)
        n108 = shared-variable "RT myRIO Target - Overlord\\Localization_Variables_r0.lvlib\\loc_flag"() -> (→"loc_flag":bool)  [unwired: 1 in, 1 out]
        n109 = local read "robot desired velocity x component\n u1 (ft/s)"() -> (w231:dbl)
        n110 = local read "robot desired velocity y component\n u2 (ft/s)"() -> (w254:dbl)
        n111 = shared-variable "RT myRIO Target - Overlord\\Localization_Variables_r0.lvlib\\loc_x"() -> (w225:dbl)  [unwired: 1 in, 1 out]
        "loc_x" <- w225
        n112 = local read "Encoder Reset"() -> (w210:bool)
        n113 = Or(x=w210, y=w212) -> (x .or. y?=w236:bool)
        n114 = case shown="True" w236 {
          tunnel: w248 -> [_ w284]
          tunnel: [1.0 w281] -> w241
          tunnel: w210 -> [_ w279]
          frame False {
          }
          frame True {
            n115 = Less?(x=w284, y=0.95) -> (x < y?=w282:bool)
            n116 = Or(x=w282, y=w279) -> (x .or. y?=w280:bool)
            n117 = case shown="True" w280 {
              tunnel: [0.85 0.0] -> w281
              frame False {
              }
              frame True {
              }
            }
          }
        }
        "Scale" <- w241
        n118 = case shown="True" w210 {
          tunnel: [1.0 0.0] -> w250
          frame False {
          }
          frame True {
          }
        }
        "Reset X Y" <- w250
        n119 = local read "track width(ft)"() -> (w230:dbl)
        n120 = Subtract(x=w225, y=w209) -> (x-y=w206:dbl)
        "x delta" <- w206
        n121 = shared-variable "RT myRIO Target - Overlord\\Localization_Variables_r0.lvlib\\loc_y"() -> (w223:dbl)  [unwired: 1 in, 1 out]
        n122 = shared-variable "RT myRIO Target - Navigation\\Navi Global Variables.lvlib\\All Stop"() -> (w275:bool)  [unwired: 1 in, 1 out]
        n123 = Add(x=w205, y=w206) -> (x+y=w202:dbl)
        "x traveled" <- w202
        n124 = Subtract(x=w223, y=w224) -> (x-y=→"y position":dbl)
        n125 = Equal To 0?(x=w241) -> (x = 0?=w274:bool)
        n126 = shared-variable "RT myRIO Target - Navigation\\Navi Global Variables.lvlib\\Start Position X"() -> (w203:dbl)  [unwired: 1 in, 1 out]
        n127 = And(x=w274, y=w275) -> (x .and. y?=w273:bool)
        n128 = shared-variable "RT myRIO Target - Navigation\\Navi Global Variables.lvlib\\Destination Reached"(w274) -> ()  [unwired: 1 in, 1 out]
        n129 = Divide(x=w202, y=1.0) -> (x/y=w200:dbl)
        n130 = Add(x=w200, y=w203) -> (x+y=→"x position camera":dbl)
        n131 = local read "loc_x"() -> (w207:dbl)
        n132 = local read "x traveled"() -> (w204:dbl)
        n133 = call "Navi R&L ENC Avg.vi"(0:w261, "encoder step sub vi input"=w260, 2:w259, 3:w258, 4:w257, 5:w256, 6:w246, "Reset X Y"=w263, 9:w262, 17:w255, 18:w218) -> ("encoder step sub vi output"=w243:dbl[])  [unwired: 8 in]
        n134 = call "Calc X & Y Position.vi"(1:w243, 4:w264, "x & y position input array"=w266, 8:w245) -> ("phi step"=w255:dbl, 3:w218, 12:w253, 18:w265)  [unwired: 11 in, 1 out]
        "phi current" <- w253
        "x traveled" <- w265
        n135 = call "Omega & Angular Velocity Calc.vi"("Phi Current"=w253, "Desired Y Velocity u2"=w254, "Desired X Velocity u1"=w231) -> ("Desired Velocity"=w226:dbl, "Phi desired"=→"Phi desired":dbl, "Omega"=w234:dbl)  [unwired: 6 in]
        "Desired Velocity" <- w226
        n136 = Merge Signals(w234, w226, w231, w230, 0.25 ("Wheel Radius")) -> (w235:dynamicdata)
        n137 = Split Signals(w235) -> (w233:dynamicdata, w232:dynamicdata, w229:dynamicdata, w228:dynamicdata)  [unwired: 5 in, 1 out]
        n138 = call "Wheel PID SetPoint.vi"("Omega"=w233, "Wheel Radius"=w228, "Track Width"=w229, "Desired Velocity"=w232) -> ("Left Side Setpoint"=→"Left Setpoint":dbl, "v left wheel"=→"v left wheel":dbl, "Right Side Setpoint"=→"Right Setpoint":dbl, "v right wheel"=→"v right wheel":dbl, "max v"=→"max v":dbl)  [unwired: 3 in]
      }
    }
    frame #4 {
      w383 = 0.0
      w392 = 0.5
      w393 = 333.3333
      # "Resets Variables back to default values"
      n139 = shared-variable "RT myRIO Target - Navigation\\Navi Global Variables.lvlib\\Destination Reached"(FALSE) -> ()  [unwired: 1 in, 1 out]
      n140 = shared-variable "RT myRIO Target - Navigation\\Navi Global Variables.lvlib\\All Stop"(FALSE) -> ()  [unwired: 1 in, 1 out]
      n141 = call <vilib>:"Set Duty Cycle and Frequency.vi"("Frequency [Hz]"=w393, "Duty Cycle"=w392, "PWM Ref In"=w391) -> ("error out"=w398:errorcluster, "PWM Ref Out"=w405:T5)  [unwired: 6 in]
      n142 = call <vilib>:"Set Duty Cycle and Frequency.vi"("Frequency [Hz]"=w393, "Duty Cycle"=w392, "PWM Ref In"=w390) -> ("error out"=w403:errorcluster, "PWM Ref Out"=w404:T5)  [unwired: 6 in]
      n143 = call <vilib>:"Set Duty Cycle and Frequency.vi"("Frequency [Hz]"=w393, "Duty Cycle"=w392, "PWM Ref In"=w389) -> ("error out"=w397:errorcluster, "PWM Ref Out"=w402:T5)  [unwired: 6 in]
      n144 = call <vilib>:"Set Duty Cycle and Frequency.vi"("Frequency [Hz]"=w393, "Duty Cycle"=w392, "PWM Ref In"=w388) -> ("error out"=w396:errorcluster, "PWM Ref Out"=w401:T5)  [unwired: 6 in]
      n145 = call <vilib>:"Set Duty Cycle and Frequency.vi"("Frequency [Hz]"=w393, "Duty Cycle"=w392, "PWM Ref In"=w387) -> ("error out"=w395:errorcluster, "PWM Ref Out"=w400:T5)  [unwired: 6 in]
      n146 = call <vilib>:"Set Duty Cycle and Frequency.vi"("Frequency [Hz]"=w393, "Duty Cycle"=w392, "PWM Ref In"=w386) -> ("error out"=w394:errorcluster, "PWM Ref Out"=w399:T5)  [unwired: 6 in]
      n147 = local write "x traveled"(w383) -> ()
      n148 = local write "y position"(w383) -> ()
      n149 = call <vilib>:"Close.vi"("error in (no error)"=w398, "PWM Ref In"=w405) -> ()  [unwired: 9 in, 1 out]
      n150 = call <vilib>:"Close.vi"("error in (no error)"=w403, "PWM Ref In"=w404) -> ()  [unwired: 9 in, 1 out]
      n151 = call <vilib>:"Close.vi"("error in (no error)"=w397, "PWM Ref In"=w402) -> ()  [unwired: 9 in, 1 out]
      n152 = call <vilib>:"Close.vi"("error in (no error)"=w396, "PWM Ref In"=w401) -> ()  [unwired: 9 in, 1 out]
      n153 = call <vilib>:"Close.vi"("error in (no error)"=w395, "PWM Ref In"=w400) -> ()  [unwired: 9 in, 1 out]
      n154 = call <vilib>:"Close.vi"("error in (no error)"=w394, "PWM Ref In"=w399) -> ()  [unwired: 9 in, 1 out]
    }
  }
